vi "Go To Position.vi"(9 "Z Position":dbl, 10 "Y Position":dbl, 11 "X Position":dbl) -> (3 "G-Code String":string)   [LabVIEW 2021]
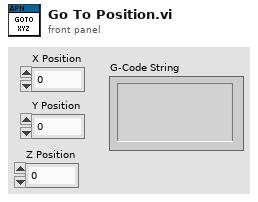
[diagram p1: front panel]
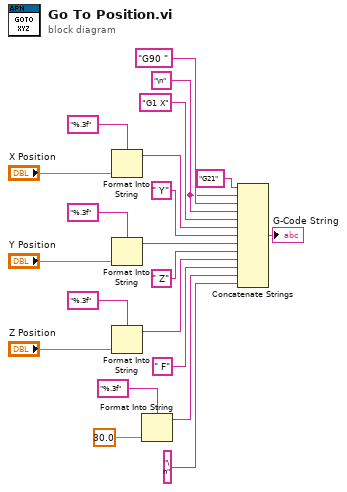
[diagram p0: block diagram]
diagram:
  w2 = "\n" ("string")
  n1 = Format Into String(format string="%.3f", "X Position") -> (resulting string=w7:string)  [unwired: 2 in, 1 out]
  n2 = Format Into String(format string="%.3f", "Y Position") -> (resulting string=w6:string)  [unwired: 2 in, 1 out]
  n3 = Format Into String(format string="%.3f", "Z Position") -> (resulting string=w3:string)  [unwired: 2 in, 1 out]
  n4 = Format Into String(format string="%.3f", 30.0 ("input 1")) -> (resulting string=w16:string)  [unwired: 2 in, 1 out]
  n5 = Concatenate Strings("G21" ("string"), w2, "G90 " ("string"), w2, "G1 X" ("string"), w7, " Y" ("string"), w6, " Z" ("string"), w3, " F" ("string"), w16, "\n" ("string")) -> (→"G-Code String":string)
